vi "subpanelStartUI.vi"(8 "error in (no error)":errorcluster, 10 "AMC*":T1, 11 "xceDataNode in":refnum<class "xceDataNode.lvclass">) -> (0 "error out":errorcluster, 2 "UI VI*":refnum<vi>, 3 "xceDataNode out":refnum<class "xceDataNode.lvclass">)   [LabVIEW 2013, in "xceDataNode.lvclass"]
doc: "Community access for the method StartUI method. Used to give access to the xceSubpanel class."
uses:
  xceDataNode.lvclass
  <vilib>/NI/AMC/Message Queue.ctl
  <vilib>/NI/AMC/Message.ctl
  <vilib>/NI/Tools/Keyed Array/KeyedArray.ctl
  <vilib>/NI/AMC/AMC.lvlib
  <vilib>/NI/Tools/Keyed Array/Tools_KeyedArray.lvlib
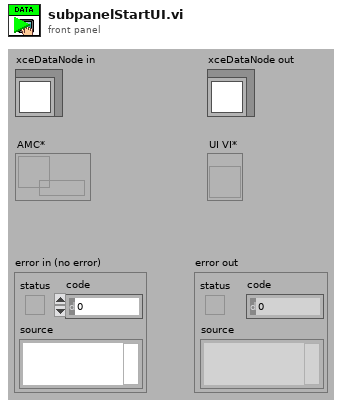
[diagram p1: front panel]
types:
  T1 = typedef "AMC.lvlib/Message Queue.ctl" = refnum<queue>
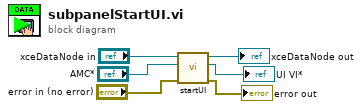
[diagram p0: block diagram]
diagram:
  n1 = call-dynamic "startUI.vi"("error in (no error)"="error in (no error)", "AMC*"="AMC*", "xceDataNode in"="xceDataNode in") -> ("error out"=→"error out":errorcluster, "UI VI*"=→"UI VI*":refnum<vi>, "xceDataNode out"=→"xceDataNode out":refnum<class "xceDataNode.lvclass">)  [unwired: 6 in]
